vi "INI Position Removed.vi"(8 "error in":errorcluster, 11 "Editor Position in":refnum<class "Editor Position.lvclass">) -> (0 "error out":errorcluster, 3 "Editor Position out":refnum<class "Editor Position.lvclass">)   [LabVIEW 2021, in "Editor Position.lvclass"]
doc: "Tests the reading of the Position and Use Position Size INI keys when the keys are removed."
uses:
  Editor Position.lvclass
  C:/Program Files/National Instruments/LabVIEW 2024/vi.lib/Astemes/LUnit/Test Case.lvclass
  <vilib>/Utility/miscctls.llb/LVRectTypeDef.ctl
  <vilib>/Astemes/LUnit/Test Case.lvclass/Test Case.ctl
  c60327dd-cdad-4b8c-8243-7f44ee2244ce.vi
  <vilib>/Astemes/LUnit/Core/LUnit Test Case/Private/Append Pass Result.vi
  <vilib>/Astemes/LUnit/Core/LUnit Test Case/Private/Append Fail Result.vi
  c60327dd-cdad-4b8c-8243-7f44ee2244ce.vi/9c5d11cd-9439-4240-a1ee-d9baace9c924.vi
  <vilib>/Astemes/LUnit/Core/LUnit Test Case/Private/Run In UI.vi
  <vilib>/Utility/error.llb/Clear Errors.vi
  <vilib>/LabVIEW Icon API/lv_icon/lv_icon.lvlib
  <vilib>/Astemes/LUnit/Test Case.lvclass
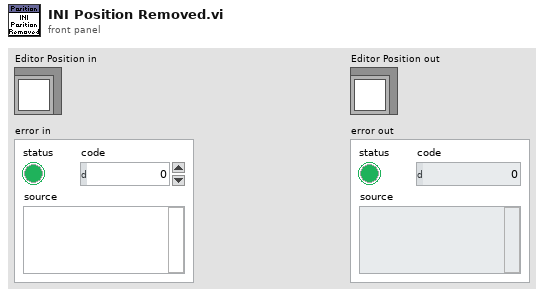
[diagram p1: front panel]
types:
  T1 = typedef "LVRectTypeDef.ctl" = cluster{"Left":i16, "Top":i16, "Right":i16, "Bottom":i16}
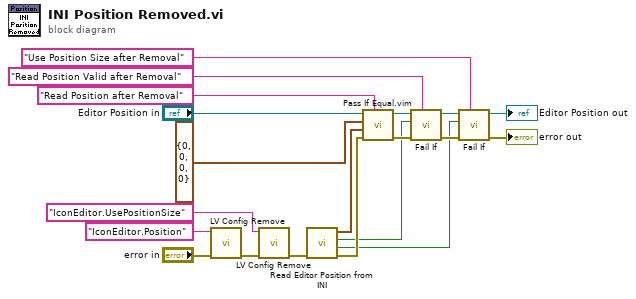
[diagram p0: block diagram]
diagram:
  n1 = call <resource>:"LV Config Remove.vi"("error in"="error in", "key"="IconEditor.Position") -> ("error out"=w17:errorcluster)  [unwired: 5 in]
  n2 = call <resource>:"LV Config Remove.vi"("error in"=w17, "key"="IconEditor.UsePositionSize") -> ("error out"=w16:errorcluster)  [unwired: 5 in]
  n3 = call <resource>:"Read Editor Position from INI.vi"("error in"=w16) -> ("error out"=w19:errorcluster, "Use Size"=w2:bool, "Bounds Valid"=w6:bool, "Window Bounds"=w7:T1)  [unwired: 7 in]
  n4 = call "Pass If Equal.vim"("Description"="Read Position after Removal", "error in (no error)"=w19, "Actual"=w7, "Expected"=T1 {"Left"=0, "Top"=0, "Right"=0, "Bottom"=0} ("Window Bounds"), "LUnit Test Case In"="Editor Position in") -> ("error out"=w20:errorcluster, "LUnit Test Case Out"=w13:refnum<class "Editor Position.lvclass">)  [unwired: 5 in]
  n5 = call <vilib>:"Fail If.vi"("Description"="Read Position Valid after Removal", "error in (no error)"=w20, "Fail?"=w6, "LUnit Test Case In"=w13) -> ("error out"=w15:errorcluster, "LUnit Test Case Out"=w3:refnum<class "Editor Position.lvclass">)  [unwired: 6 in]
  n6 = call <vilib>:"Fail If.vi"("Description"="Use Position Size after Removal", "error in (no error)"=w15, "Fail?"=w2, "LUnit Test Case In"=w3) -> ("error out"=→"error out":errorcluster, "LUnit Test Case Out"=→"Editor Position out":refnum<class "Editor Position.lvclass">)  [unwired: 6 in]
